vi "AVS_Switch_channel.vi"(8 "error in (no error) 3":errorcluster, 9 "AVS Excitation":i8, 10 "AVS Channel":i8, 11 "AVS-VISA":refnum<visa-resource-name>) -> (0 "error out (no error) 2":errorcluster, 3 "dup VISA-AVS":refnum<visa-resource-name>)   [LabVIEW 2018]
uses:
  Instrument_Setup.vi
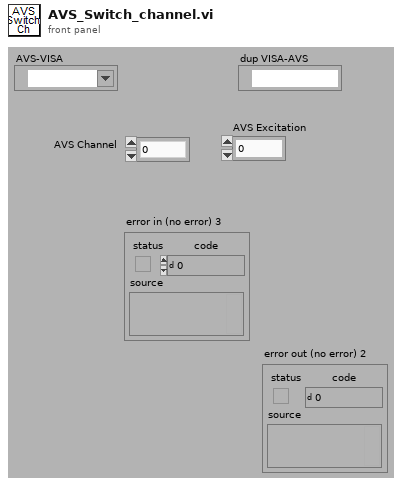
[diagram p1: front panel]
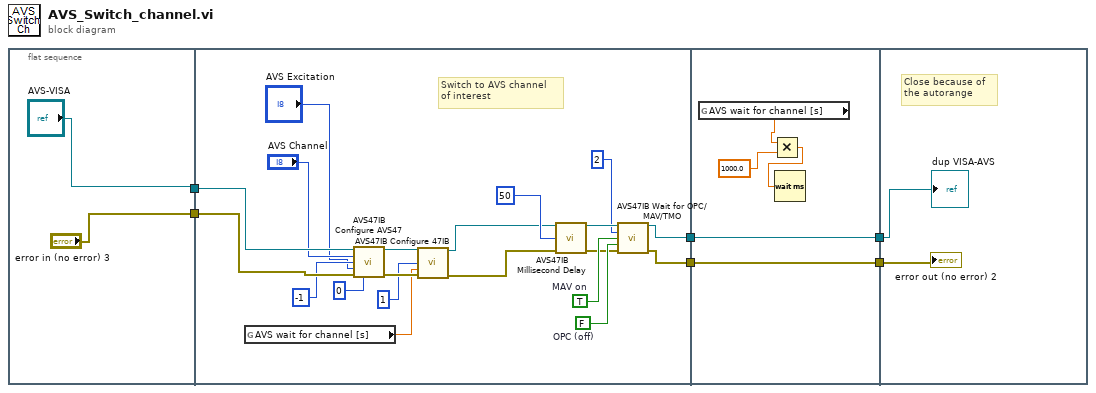
[diagram p0: block diagram]
diagram:
  n1 = flat-sequence {
    tunnel: ["AVS-VISA"] -> w6
    tunnel: ["error in (no error) 3"] -> w5
    tunnel: [w22] -> w4
    tunnel: [w21] -> w2
    tunnel: w6 -> [w20]
    tunnel: w5 -> [w19]
    tunnel: w4 -> [w33]
    tunnel: [w33] -> w3
    tunnel: w2 -> [w32]
    tunnel: [w32] -> w1
    tunnel: w3 -> [w34]
    tunnel: w1 -> [w35]
    frame #0 {
    }
    frame #1 {
      w26 = FALSE  # OPC (off)
      w27 = TRUE  # MAV on
      # "Switch to AVS channel \nof interest"
      n2 = global read "Instrument_Setup.vi" "AVS wait for channel [s]"() -> (w9:dbl)
      n3 = call "AVS47IB Configure AVS47.vi"("VISA session"=w20, "CHANNEL (-1:no change )"="AVS Channel", "RANGE  (-1:no change)"=i8 -1 ("DISPLAY (-1:no change)"), "EXCITATION (-1:no change)"="AVS Excitation", "error in (no error)"=w19, "DISPLAY (-1:no change)"=i8 0) -> ("dup VISA session"=w15:refnum<visa-resource-name>, "error out"=w14:errorcluster)  [unwired: 8 in]
      n4 = call "AVS47IB Configure 47IB.vi"("VISA session"=w15, "Autoranging Enabled (-1:no change)"=i8 1, "Stabilisation Delay (-1:no change)"=w9, "error in (no error)"=w14) -> ("dup VISA session"=w13:refnum<visa-resource-name>, "error out"=w12:errorcluster)  [unwired: 10 in]
      n5 = call "AVS47IB Millisecond Delay.vi"("VISA session"=w13, "Delay (50 ms)"=u32 50, "error in (no error)"=w12) -> ("dup VISA session"=w25:refnum<visa-resource-name>, "error out"=w24:errorcluster)  [unwired: 11 in]
      n6 = call "AVS47IB Wait for OPC/MAV/TMO.vi"("VISA session"=w25, "Timeout (2 sec)"=i16 2, "MAV (on)"=w27, "OPC (off)"=w26, "error in (no error)"=w24) -> ("dup VISA session"=w22:refnum<visa-resource-name>, "error out"=w21:errorcluster)  [unwired: 8 in, 1 out]
    }
    frame #2 {
      n7 = global read "Instrument_Setup.vi" "AVS wait for channel [s]"() -> (w31:dbl)
      n8 = Multiply(x=w31, y=1000.0) -> (x*y=w29:dbl)
      n9 = Wait (ms)(milliseconds to wait=w29) -> ()  [unwired: 1 out]
    }
    frame #3 {
      # "Close because of \nthe autorange"
      "error out (no error) 2" <- w35
      "dup VISA-AVS" <- w34
    }
  }
